vi "AssertValueByFocusNamePath.vi"(0 "VI Reference In":refnum<vi>, 1 "Test Label":string, 2 "delimiter (>>)":string=">>", 3 "Assert Only? (F)":bool, 5 "Control Path":string, 7 "Focus Item Path":string, 11 "Error In":errorcluster, 12 "Assert Interval(10 ms)":u32=10, 13 "Timeout(5 sec)":dbl=5.0) -> (4 "VI Reference Out":refnum<vi>, 6 "Asserted Value":string, 15 "Error Out":errorcluster)   [LabVIEW 2016, in "Drona.lvlib" / "AssertControlValue.lvlib" / "AssertTree.lvlib"]
doc: "Asserts if the focus item name given as hierarchical path on tree controls is equal.\n\nHierarchical path represent their corresponding parents of an item from its origin. Use the delimiters '>>' between each hierarchy in the path.\n\nFor example to select the item 'Child3', give the hierarchical path as \"<b>Parent1</b>(top level parent in tree)<b>>>Child1</b>(children for parent1)<b>>>Child2</b>(children for child1)<b>>>Child3</b>(children for child2)\"\nThe input control name is given as a string , incase of path, use delimiters inbetween the path.\nThis VI gets the value of the control, untill the value is equal to the input value."
uses:
  AssertTree.lvlib
  Get/GetControlRef/GetControlRefByPath.vi
  <vilib>/Utility/error.llb/Error Cluster From Error Code.vi
  <vilib>/addons/_JKI Toolkits/Caraya/classes/Assert/Assert Equal Value_Variant.vi
  <vilib>/ErrorRing/Error Ring.xnode
  Get/GetControlRef/GetControlRef.lvlib
  <vilib>/addons/_JKI Toolkits/Caraya/classes/Assert/Assert.lvclass
  Drona.lvlib
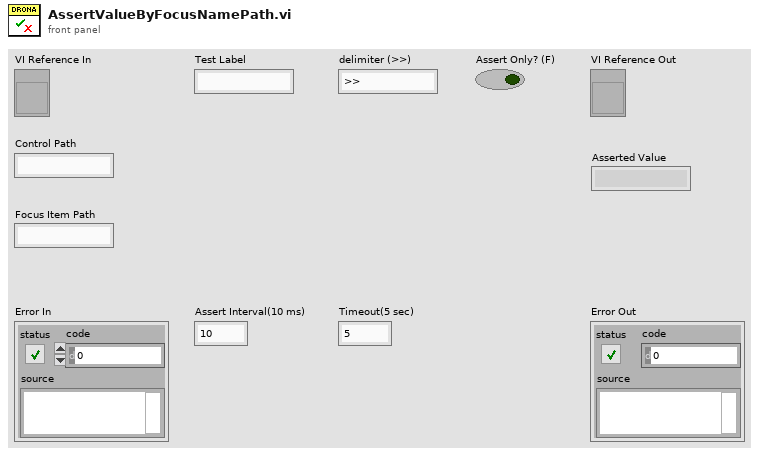
[diagram p1: front panel]
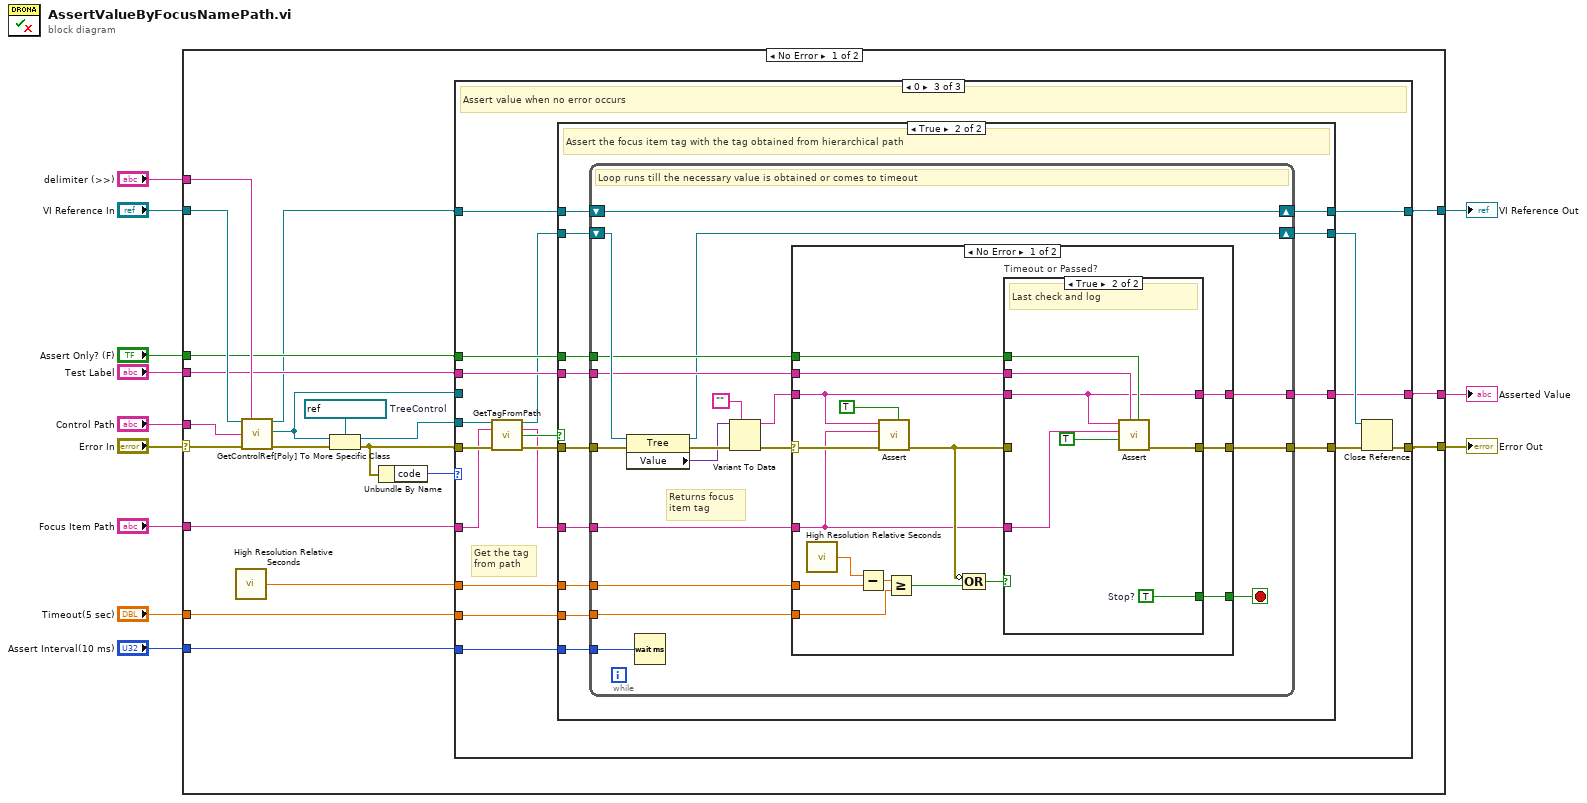
[diagram p0: block diagram]
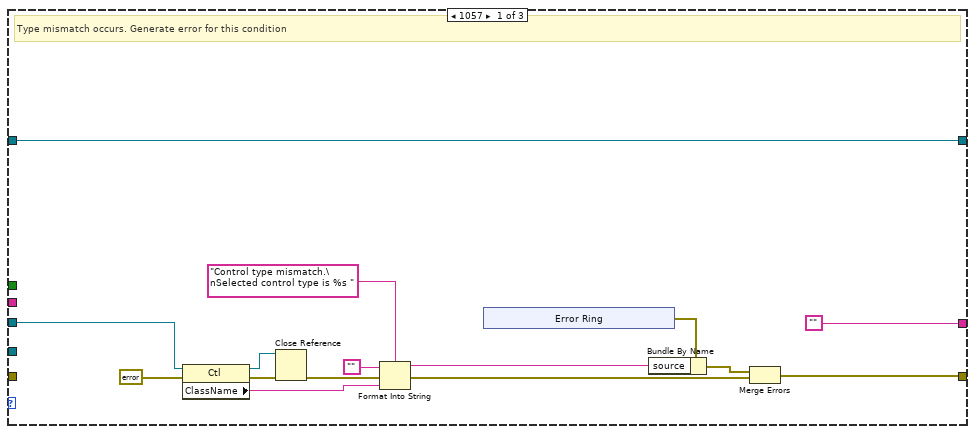
[diagram p2: hidden frame]
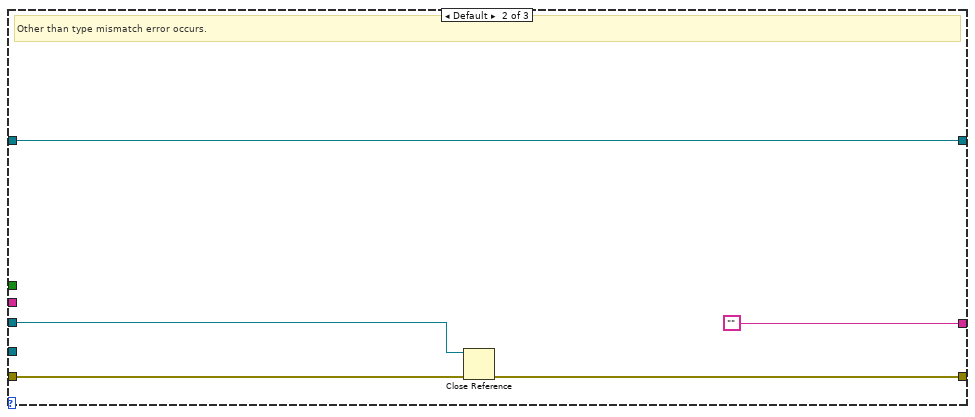
[diagram p3: hidden frame]
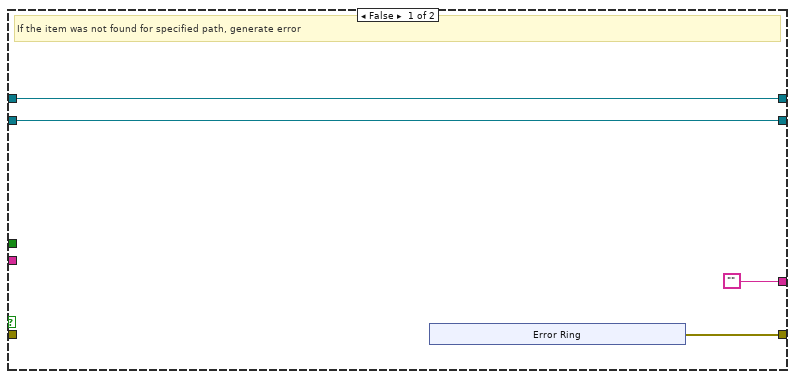
[diagram p4: hidden frame]
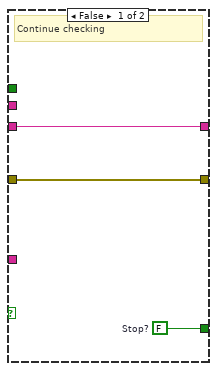
[diagram p5: hidden frame]
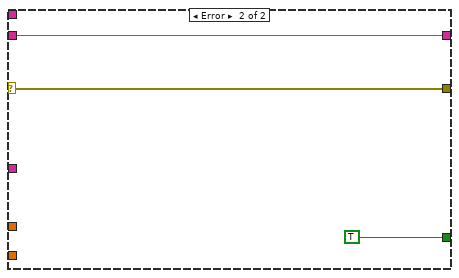
[diagram p6: hidden frame]
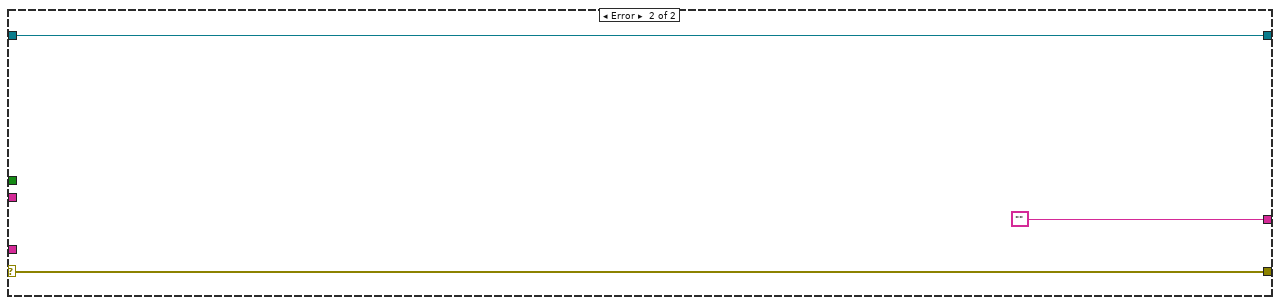
[diagram p7: hidden frame]
diagram:
  n1 = case shown="No Error" "Error In" {
    selector: "Error In" -> [w32 w147]
    tunnel: "Timeout(5 sec)" -> [w18 _]
    tunnel: [w14 w146] -> w11
    tunnel: "Focus Item Path" -> [w20 _]
    tunnel: [w15 w147] -> w10
    tunnel: "Assert Interval(10 ms)" -> [w17 _]
    tunnel: "Test Label" -> [w23 _]
    tunnel: "VI Reference In" -> [w31 w146]
    tunnel: "Control Path" -> [w30 _]
    tunnel: "delimiter (>>)" -> [w28 _]
    tunnel: "Assert Only? (F)" -> [w22 _]
    tunnel: [w16 ""] -> w1
    frame No Error {
      w27 = refnum<vi> refnum  # TreeControl
      n2 = call <vilib>:"High Resolution Relative Seconds.vi"() -> ("relative seconds"=w19:dbl)
      n3 = call-poly "GetControlRef[Poly].vi"("VI Reference In"=w31, "delimiter (>>)"=w28, "Control Path"=w30, "error In"=w32) -> ("VI Reference Out"=w21:refnum<vi>, "Ctl Refnum"=w24:refnum<vi>, "error out"=w29:errorcluster)  [unwired: 9 in]
      n4 = To More Specific Class(target class=w27, reference=w24, error in=w29) -> (specific class reference=w25:refnum<vi>, error out=w26:errorcluster)
      n5 = Unbundle By Name(w26) -> ("code"=w13:i32)
      n6 = case shown="0" w13 {
        tunnel: w18 -> [_ _ w75]
        tunnel: [w47 w57 w74] -> w14
        tunnel: w20 -> [_ _ w60]
        tunnel: w17 -> [_ _ w72]
        tunnel: w23 -> [_ _ w71]
        tunnel: w19 -> [_ _ w70]
        tunnel: w21 -> [w47 w57 w69]
        tunnel: [w34 w54 w68] -> w15
        tunnel: w22 -> [_ _ w66]
        tunnel: ["" "" w65] -> w16
        tunnel: w26 -> [_ w56 w64]
        tunnel: w25 -> [_ _ w61]
        tunnel: w24 -> [w33 w53 _]
        frame 1057 {
          # "Type mismatch occurs. Generate error for this condition"
          n7 = property class="Ctl"(reference=w33, error in=errorcluster {"status"=FALSE, "code"=0, "source"=""} ("error out")) -> (reference out=w35:refnum<vi>, error out=w45:errorcluster, "ClassName"=w42:string)
          n8 = Close Reference(reference=w35, error in (no error)=w45) -> (error out=w36:errorcluster)
          n9 = Format Into String(format string="Control type mismatch.\nSelected control type is %s ", initial string="", error in=w36, w42) -> (resulting string=w39:string, error out=w37:errorcluster)
          n10 = xnode "Error Ring"() -> ("error out"=w40:errorcluster)
          n11 = Bundle By Name(cluster=w40, "source"=w39) -> (w38:errorcluster)
          n12 = Merge Errors(w38, w37) -> (w34:errorcluster)
        }
        frame Default {
          # "Other than type mismatch error occurs."
          n13 = Close Reference(reference=w53, error in (no error)=w56) -> (error out=w54:errorcluster)
        }
        frame 0 {
          # "Get the tag \nfrom path"
          # "Assert value when no error occurs"
          n14 = call "GetTagFromPath.vi"("Tree Ref In"=w61, "Hierarchical Path"=w60, "Error In"=w64) -> ("Tree Ref Out"=w58:refnum<vi>, "Item Tag"=w59:string, "Item Found?"=w62:bool, "Error Out"=w63:errorcluster)  [unwired: 9 in]
          n15 = case shown="True" w62 {
            tunnel: w75 -> [_ w97]
            tunnel: [w79 w96] -> w74
            tunnel: [w76 w95] -> w73
            tunnel: w72 -> [_ w94]
            tunnel: w71 -> [_ w93]
            tunnel: w70 -> [_ w92]
            tunnel: w69 -> [w79 w91]
            tunnel: [w78 w90] -> w67
            tunnel: w66 -> [_ w89]
            tunnel: ["" w88] -> w65
            tunnel: w59 -> [_ w87]
            tunnel: w58 -> [w78 w85]
            tunnel: w63 -> [_ w86]
            frame False {
              # "If the item was not found for specified path, generate error"
              n16 = xnode "Error Ring"() -> ("error out"=w76:errorcluster)
            }
            frame True {
              # "Assert the focus item tag with the tag obtained from hierarchical path"
              n17 = while {
                tunnel: w87 -> [w103]
                tunnel: w97 -> [w114]
                tunnel: w92 -> [w115]
                tunnel: w86 -> [w109]
                tunnel: [w112] -> w95
                tunnel: w94 -> [w110]
                tunnel: w93 -> [w106]
                shift-right: [w107] -> w96
                shift-left: w91 -> [w107]
                shift-right: [w98] -> w90
                shift-left: w85 -> [w108]
                tunnel: w89 -> [w105]
                tunnel: [w104] -> w88
                stop <- w113 stop-if-true
                # "Returns focus \nitem tag"
                # "Loop runs till the necessary value is obtained or comes to timeout"
                n18 = property on="Property Node" class="Tree"(reference=w108, error in=w109) -> (reference out=w98:refnum<vi>, error out=w111:errorcluster, "Value"=w101:variant)
                n19 = Wait (ms)(milliseconds to wait=w110) -> ()  [unwired: 1 out]
                n20 = Variant To Data(error in=w111, type="", Variant=w101) -> (data=w99:string, error out=w102:errorcluster)
                n21 = case shown="No Error" w102 {
                  selector: w102 -> [w127 w144]
                  tunnel: w115 -> [w131 _]
                  tunnel: w114 -> [w128 _]
                  tunnel: [w118 TRUE] -> w113
                  tunnel: [w119 w144] -> w112
                  tunnel: w103 -> [w120 _]
                  tunnel: w99 -> [w121 w142]
                  tunnel: w106 -> [w126 _]
                  tunnel: w105 -> [w117 _]
                  tunnel: [w116 w142] -> w104
                  frame No Error {
                    n22 = call <vilib>:"High Resolution Relative Seconds.vi"() -> ("relative seconds"=w130:dbl)
                    n23 = Subtract(x=w130, y=w131) -> (x-y=w129:dbl)
                    n24 = call-poly <vilib>:"Assert.vi"("Assert Only? (F)"=TRUE, "error in (no error)"=w127, "Y"=w120, "X"=w121) -> ("error out"=w124:errorcluster)  [unwired: 7 in]
                    n25 = Greater Or Equal?(x=w129, y=w128) -> (x >= y?=w125:bool)
                    n26 = Compound Arithmetic op=OR(invert w124, w125) -> (w123:bool)
                    n27 = case "Timeout or Passed?" shown="True" w123 {
                      tunnel: w124 -> [w134 _]
                      tunnel: w120 -> [_ w137]
                      tunnel: w121 -> [w132 w136]
                      tunnel: w126 -> [_ w141]
                      tunnel: [w134 w140] -> w119
                      tunnel: [w133 w139] -> w118
                      tunnel: w117 -> [_ w138]
                      tunnel: [w132 w136] -> w116
                      frame False {
                        w133 = FALSE  # Stop?
                        # "Continue checking"
                      }
                      frame True {
                        w139 = TRUE  # Stop?
                        # "Last check and log"
                        n28 = call-poly <vilib>:"Assert.vi"("Assert Only? (F)"=w138, "Label"=w141, "Register with caller test (F)"=TRUE, "Y"=w137, "X"=w136) -> ("error out"=w140:errorcluster)  [unwired: 6 in]
                      }
                    }
                  }
                  frame Error {
                  }
                }
              }
            }
          }
          n29 = Close Reference(reference=w67, error in (no error)=w73) -> (error out=w68:errorcluster)
        }
      }
    }
    frame Error {
    }
  }
  "Error Out" <- w10
  "VI Reference Out" <- w11
  "Asserted Value" <- w1
